vi "c Spark Get Serial Number.vi"(8 "error in (no error)":errorcluster, 10 "serialNumber":u32[](array[numeric])=[0, 0, 0], 11 "handle":T1) -> (0 "error out":errorcluster, 1 "function return":T2, 2 "serialNumber out":u32[](array[numeric]), 3 "handle out":T1)   [LabVIEW 2023, in "REVLibDriver.lvlib"]
doc: "c_REVLib_ErrorCode c_Spark_GetSerialNumber(c_Spark_handle handle,\n unsigned __int32* serialNumber[3]);"
uses:
  <vilib>/REVLibDriver5/REVLibDriver.lvlib
  lib/libREVLibDriver.so
  <vilib>/Custom Controls/c_Spark_handle.ctl
  <vilib>/REVLibDriver5/subvi/RevLibError.ctl
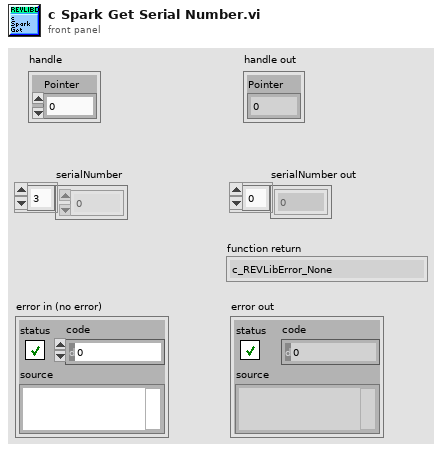
[diagram p1: front panel]
types:
  T1 = typedef "REVLibDriver.lvlib/c_Spark_handle.ctl" = cluster{"Pointer":u64}
  T2 = typedef "REVLibDriver.lvlib/RevLibError.ctl" = enum16{"c_REVLibError_None", "c_REVLibError_General", "c_REVLibError_CANTimeout", "c_REVLibError_NotImplemented", "c_REVLibError_HAL", "c_REVLibError_CantFindFirmware", "c_REVLibError_FirmwareTooOld", "c_REVLibError_FirmwareTooNew", "c_REVLibError_ParamInvalidID", "c_REVLibError_ParamMismatchType", "c_REVLibError_ParamAccessMode", "c_REVLibError_ParamInvalid", "c_REVLibError_ParamNotImplementedDeprecated", "c_REVLibError_FollowConfigMismatch", "c_REVLibError_Invalid", "c_REVLibError_SetpointOutOfRange", "c_REVLibError_Unknown", "c_REVLibError_CANDisconnected", "c_REVLibError_DuplicateCANId", "c_REVLibError_InvalidCANId", "c_REVLibError_SparkMaxDataPortAlreadyConfiguredDifferently", "c_REVLibError_SparkFlexBrushedWithoutDock", "c_REVLibError_NumCodes"}
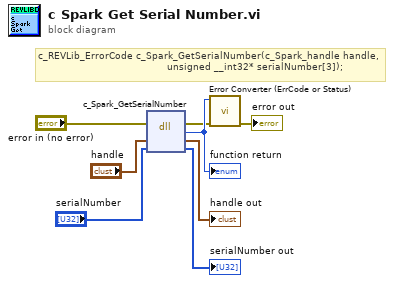
[diagram p0: block diagram]
diagram:
  # "c_REVLib_ErrorCode c_Spark_GetSerialNumber(c_Spark_handle handle,\n                                           unsigned __int32* serialNumber[3]);"
  n1 = dll-call lib="home/systemcore/natinst/lib/libREVLibDriver.so" fn="c_Spark_GetSerialNumber"(error in="error in (no error)", "handle"="handle", "serialNumber"="serialNumber") -> (error out=w2:errorcluster, "return type"=w8:u32, "handle"=→"handle out":T1, "serialNumber"=→"serialNumber out":u32[])  [unwired: 2 in, 1 out]
  "function return" <- w8
  n2 = call <vilib>:"Error Converter (ErrCode or Status).vi"("error in (no error)"=w2, "error code"=w8) -> ("error out"=→"error out":errorcluster)  [unwired: 9 in]
